vi "Write Internal FPGA FIFOs.vi"(11 "Filtered Array In":T1=[0.0, 0.0, 0.0, 0.0, 0.0, 0.0, 0.0, 0.0, 0.0, 0.0, 0.0, 0.0, 0.0, 0.0, 0.0, 0.0, 0.0, 0.0, 0.0, 0.0, 0.0, 0.0, 0.0, 0.0, 0.0, 0.0, 0.0, 0.0, 0.0, 0.0, 0.0, 0.0, 0.0, 0.0, 0.0, 0.0, 0.0, 0.0, 0.0, 0.0, 0.0, 0.0, 0.0, 0.0, 0.0, 0.0, 0.0, 0.0, 0.0, 0.0, 0.0, 0.0, 0.0, 0.0] format="%_6g") -> (2 "Timout":bool, 3 "Dump Resistor Voltage":T2 format="%.3f")   [LabVIEW 2022 SP3]
doc: "Author: Scott Hannahs <sth@magnet.fsu.edu>\nCopyright 2018 Florida State University, All rights reserved."
uses:
  SCH Data Controls/SCH Data 2 RT.ctl
  SCH Data Controls/SCH Data 2 RT Array.ctl
  <vilib>/rvi/Emulation/niFpgaEmulationIsFPGAContextNoSignature.vi
  <vilib>/rvi/Emulation/niFpgaSctlEmulationGetInTimedLoop.vi
  <vilib>/rvi/errors/niFpgaSetErrorForExecOnDevCompSimple.vi
  <vilib>/rvi/eio/common/nirviEmuReportErrorAndStop.vi
  <vilib>/rvi/DataTransferAndStorage/Container/Common/niFpgaContainerGetUniqueNameForEmu.vi
  <vilib>/rvi/FIFO/Fifo_Resource/nirvififoEmulationSetSize.vi
  <vilib>/rvi/FIFO/Fifo_Resource/nirviFifoEmulationQueueMgr.vi
  <instcachedir>/0/nirviFifoEmulationQueueMgr_E5CAEC123FF24DC58D834DCA3CDAA9B5.lvgen/nirviFifoEmulationQueueMgr_E5CAEC123FF24DC58D834DCA3CDAA9B5_001.vi
  <vilib>/rvi/FIFO/Fifo_Resource/nirvififoEmulationDetermineInputValidOut.vi
  <vilib>/rvi/FIFO/Fifo_Resource/nirvififoEmulationCreateLock.vi
  <vilib>/rvi/Emulation/niFpgaProcessEmulError.vi
  <vilib>/rvi/FIFO/Fifo_Resource/nirvififoEmulationObtainLock.vi
  <vilib>/rvi/FIFO/Fifo_Resource/nirvififoEmulationReleaseLock.vi
  <vilib>/rvi/occurrence/nirviWaitOnOccurrenceBase.vi
  <vilib>/rvi/errors/nirviReportUnexpectedCaseInternalError.vi
  <vilib>/rvi/errors/nirviReportUnexpectedCaseInternalError (U32).vi
  <instcachedir>/0/nirviFifoEmulationQueueMgr_E5CAEC123FF24DC58D834DCA3CDAA9B5.lvgen/nirviFifoEmulationQueueMgr_E5CAEC123FF24DC58D834DCA3CDAA9B5_002.vi
  <instcachedir>/0/nirviFifoEmulationQueueMgr_E5CAEC123FF24DC58D834DCA3CDAA9B5.lvgen/nirviFifoEmulationQueueMgr_E5CAEC123FF24DC58D834DCA3CDAA9B5_003.vi
  <instcachedir>/0/nirviFifoEmulationQueueMgr_E5CAEC123FF24DC58D834DCA3CDAA9B5.lvgen/nirviFifoEmulationQueueMgr_E5CAEC123FF24DC58D834DCA3CDAA9B5_004.vi
  <instcachedir>/0/nirviFifoEmulationQueueMgr_E5CAEC123FF24DC58D834DCA3CDAA9B5.lvgen/nirviFifoEmulationQueueMgr_E5CAEC123FF24DC58D834DCA3CDAA9B5_005.vi
  <vilib>/rvi/DataTransferAndStorage/Container/XNode/niFpgaContainer.xnode
  <vilib>/rvi/FIFO/Fifo_Resource/nirvififoEmulationWrite.vi
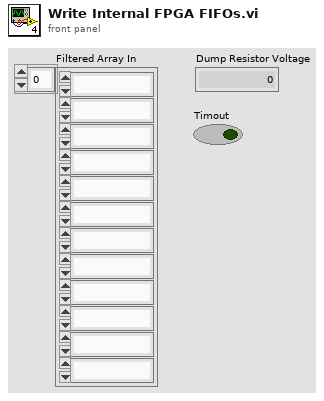
[diagram p1: front panel]
types:
  T1 = typedef "SCH Data 2 RT Array.ctl" = T2[]
  T2 = typedef "SCH Data 2 RT.ctl" = fxp<+/-,38,12>
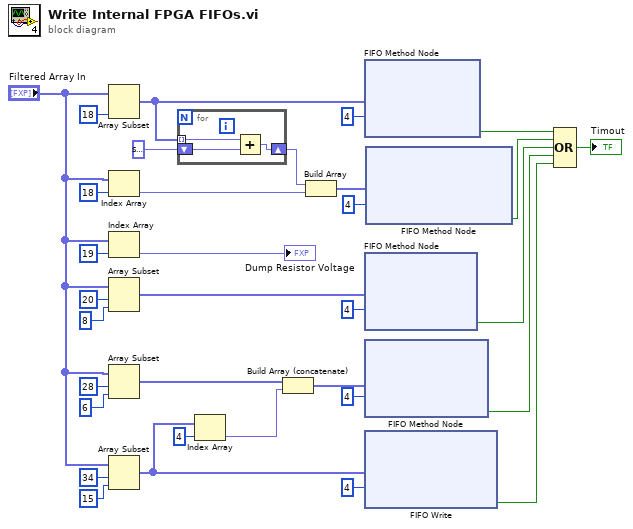
[diagram p0: block diagram]
diagram:
  n1 = Array Subset(array="Filtered Array In", length=18) -> (w12:T2[])  [unwired: 1 in]
  n2 = Index Array(array="Filtered Array In", index=18) -> (element=w15:T2)
  n3 = Index Array(array="Filtered Array In", index=19) -> (element=→"Dump Resistor Voltage":T2)
  n4 = Array Subset(array="Filtered Array In", index=20, length=8) -> (w16:T2[])
  n5 = Array Subset(array="Filtered Array In", index=28, length=6) -> (w17:T2[])
  n6 = Array Subset(array="Filtered Array In", index=34, length=15) -> (w32:T2[])
  n7 = for {
    tunnel: w12 -> [w35] mode=indexing
    shift-right: [w34] -> w14
    shift-left: T2 0.0 ("Numeric") -> [w36]
    n8 = Add(x=w35, y=w36) -> (x+y=w34:T2)
  }
  n9 = Index Array(array=w32, index=4) -> (element=w31:T2)
  n10 = Build Array (concatenate)(w17, w31) -> (w30:T2[])
  n11 = Build Array(w14, w15) -> (w3:T2[])
  n12 = xnode ("FIFO Method Node")("Element"=w12, "Timeout"=4) -> ("Timed Out?"=w22:bool)  [unwired: 1 in, 1 out]
  n13 = xnode ("FIFO Method Node")("Element"=w16, "Timeout"=4) -> ("Timed Out?"=w26:bool)  [unwired: 1 in, 1 out]
  n14 = xnode ("FIFO Method Node")("Element"=w30, "Timeout"=4) -> ("Timed Out?"=w27:bool)  [unwired: 1 in, 1 out]
  n15 = xnode ("FIFO Write")("Element"=w32, "Timeout"=4) -> ("Timed Out?"=w28:bool)  [unwired: 1 in, 1 out]
  n16 = xnode ("FIFO Method Node")("Element"=w3, "Timeout"=4) -> ("Timed Out?"=w25:bool)  [unwired: 1 in, 1 out]
  n17 = Compound Arithmetic op=OR(w22, w25, w26, w27, w28) -> (→"Timout":bool)
